vi "RMDiscardBead.vi"(10 "beadIndex":i32, 11 "ResultManager":T1) -> (3 "ResultManager (out)":T1)   [LabVIEW 2011]
uses:
  ResultManagerInstance.ctl
  QTrkDLL.vi
panel:
  out "error out":errorcluster
  in  "error in (no error)":errorcluster
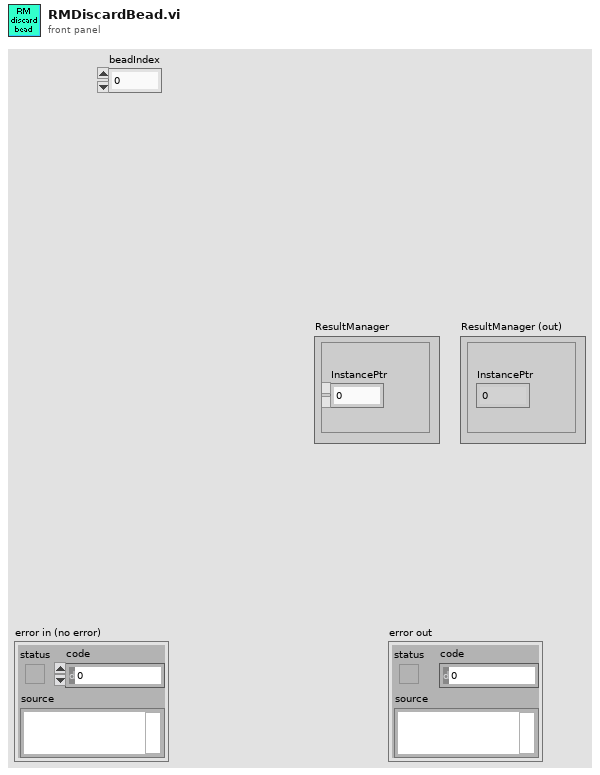
[diagram p1: front panel]
types:
  T1 = typedef "ResultManagerInstance.ctl" = cluster{"InstancePtr":u64}
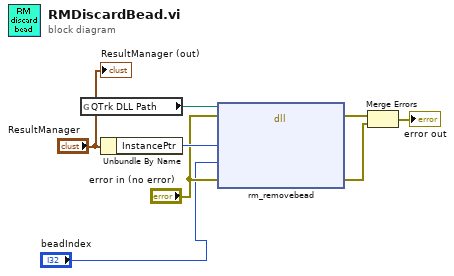
[diagram p0: block diagram]
diagram:
  n1 = global read "QTrkDLL.vi" "QTrk DLL Path"() -> (w6:path)
  n2 = Unbundle By Name("ResultManager") -> ("InstancePtr"=w7:u64)
  n3 = dll-call lib="D:/jcnossen1/cudaqi-tracker/qtrk/lv/qtrk-labview.dll" fn="rm_removebead"(path in=w6, error in="error in (no error)", "resultmanager"=w7, "beadIndex"="beadIndex", "error"="error in (no error)") -> (error out=w4:errorcluster, "error"=w3:errorcluster)  [unwired: 4 in, 1 out]
  n4 = Merge Errors(w4, w3) -> (→"error out":errorcluster)
  "ResultManager (out)" <- "ResultManager"
